vi "Auto Iterate.vi"(11 "Auto Iterate in":refnum<class "Auto Iterate.lvclass">) -> (3 "Auto Iterate out":refnum<class "Auto Iterate.lvclass">)   [LabVIEW 2021, in "Hello World Event.lvlib" / "Auto Iterate Msg Strategy.lvlib" / "Auto Iterate.lvclass"]
uses:
  Auto Iterate.lvclass
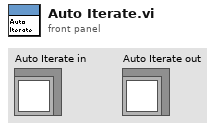
[diagram p1: front panel]
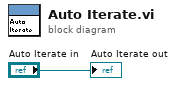
[diagram p0: block diagram]
diagram:
  "Auto Iterate out" <- "Auto Iterate in"
